vi "Write Paired Module UID.vi"(8 "error in (no error)":errorcluster, 10 "Paired Module UID":string, 11 "E2E editor node in":refnum<data-value>) -> (0 "error out":errorcluster, 3 "E2E editor node out":refnum<data-value>)   [LabVIEW 2015, in "E2E Tag Exchange editor node.lvclass"]
uses:
  E2E Tag Exchange editor node.lvclass
  module/configuration/E2E Tag Exchange configuration.lvclass
  module/configuration/E2E Tag Exchange configuration.lvclass/E2E Tag Exchange configuration.ctl
  <vilib>/NI/Configuration Framework/serializable configuration/NISE_CEF_serializable configuration.lvclass
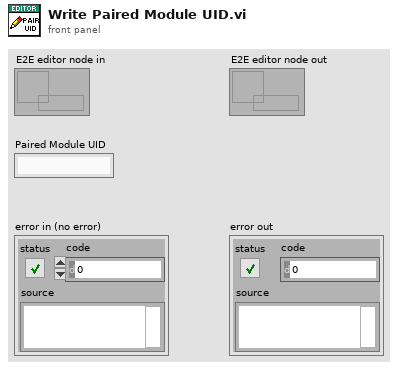
[diagram p1: front panel]
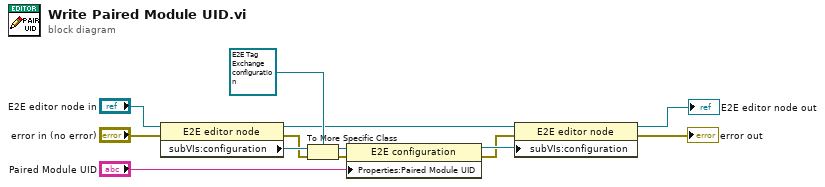
[diagram p0: block diagram]
diagram:
  n1 = property class="E2E editor node"(reference="E2E editor node in", error in="error in (no error)") -> (reference out=w6:refnum<data-value>, error out=w11:errorcluster, "subVIs:configuration"=w12:refnum<class "NISE_CEF_serializable configuration.lvclass">)
  n2 = To More Specific Class(target class=refnum<class "E2E Tag Exchange configuration.lvclass"> refnum ("E2E configuration"), reference=w12, error in=w11) -> (specific class reference=w8:refnum<class "E2E Tag Exchange configuration.lvclass">, error out=w9:errorcluster)
  n3 = property class="E2E configuration"(reference=w8, error in=w9, "Properties:Paired Module UID"="Paired Module UID") -> (reference out=w5:refnum<class "E2E Tag Exchange configuration.lvclass">, error out=w4:errorcluster)
  n4 = property class="E2E editor node"(reference=w6, error in=w4, "subVIs:configuration"=w5) -> (reference out=→"E2E editor node out":refnum<data-value>, error out=→"error out":errorcluster)
